vi "List Tables.vi"(8 "error in (no error)":errorcluster, 11 "Data.PG":refnum<class "LV-Data.PGSQL.lvclass">) -> (0 "error out":errorcluster, 1 "Table Paths":string[](array[string]), 2 "Table Names":string[](array[string]), 3 "Data.PG":refnum<class "LV-Data.PGSQL.lvclass">)   [LabVIEW 2019, in "LV-Data.PGSQL.lvclass"]
uses:
  LV-Data.PGSQL.lvclass
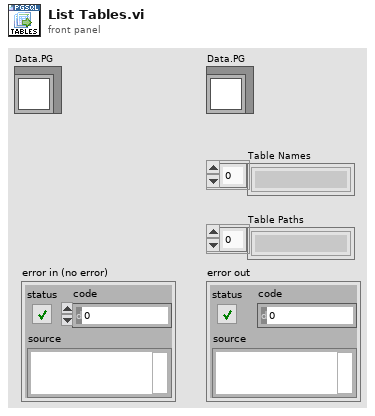
[diagram p1: front panel]
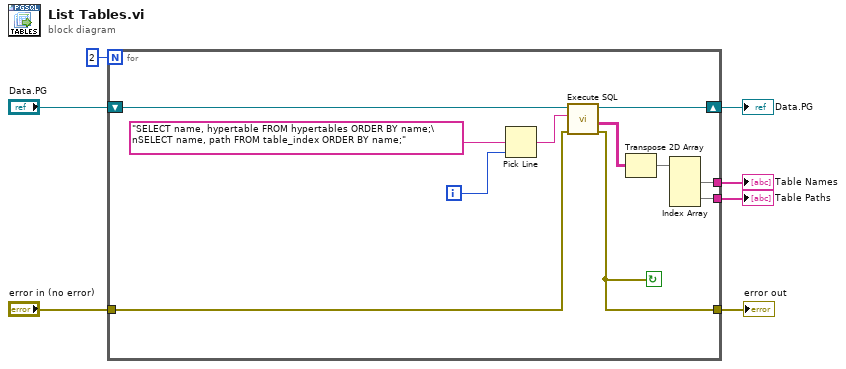
[diagram p0: block diagram]
diagram:
  n1 = for {
    N: 2 -> [_]
    tunnel: [w18] -> w7
    tunnel: [w17] -> w6
    shift-right: [w14] -> w4
    shift-left: "Data.PG" -> [w15]
    tunnel: "error in (no error)" -> [w13]
    tunnel: [w12] -> w2
    i -> [w9]
    stop <- w12 continue-if-true
    n2 = Pick Line(multi-line string="SELECT name, hypertable FROM hypertables ORDER BY name;\nSELECT name, path FROM table_index ORDER BY name;" ("command"), line index=w9) -> (output string=w10:string)  [unwired: 1 in]
    n3 = call "Execute SQL.vi"("error in"=w13, "SQL"=w10, "LV-Data.PGSQL"=w15) -> ("error out"=w12:errorcluster, "Result"=w8:string[][], "LV-Data.PGSQL out"=w14:refnum<class "LV-Data.PGSQL.lvclass">)  [unwired: 5 in, 1 out]
    n4 = Transpose 2D Array(2D array=w8) -> (transposed array=w16:string[][])
    n5 = Index Array(array=w16) -> (element #1=w17:string[], element #2=w18:string[])  [unwired: 4 in]
  }
  "Table Paths" <- w7
  "Table Names" <- w6
  "error out" <- w2
  "Data.PG" <- w4
